vi "Calc Profile Data Size.vi"(4 "Profile Info":T1) -> (1 "Profile Data Size in U32":u32)   [LabVIEW 2014]
uses:
  Public/Clusters/Profile Info.ctl
  Keyence LJ-V7000.lvlib
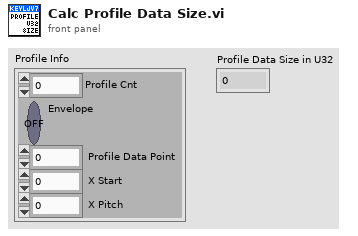
[diagram p1: front panel]
types:
  T1 = typedef "Keyence LJ-V7000.lvlib/Profile Info.ctl" = cluster{"Profile Cnt":u8, "Envelope":bool, " Profile Data Point":u16, " X Start":i32, " X Pitch":i32}
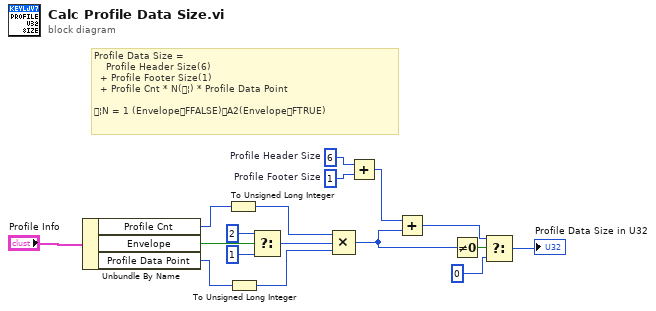
[diagram p0: block diagram]
diagram:
  w2 = u32 1  # Profile Footer Size
  w3 = u32 6  # Profile Header Size
  # "Profile Data Size =\n    Profile Header Size(6)\n  + Profile Footer Size(1)\n  + Profile Cnt * N(¦) * Profile Data Point\n\n¦N = 1 (EnvelopeFFALSE)A2(EnvelopeFTRUE)"
  n1 = Unbundle By Name("Profile Info") -> ("Profile Cnt"=w6:u8, "Envelope"=w5:bool, "Profile Data Point"=w4:u16)
  n2 = To Unsigned Long Integer(number=w6) -> (unsigned 32bit integer=w14:u32)
  n3 = To Unsigned Long Integer(number=w4) -> (unsigned 32bit integer=w12:u32)
  n4 = Select(t=u32 2, s=w5, f=u32 1) -> (s? t:f=w13:u32)
  n5 = Compound Arithmetic op=MULTIPLY(w14, w13, w12) -> (w9:u32)
  n6 = Add(x=w3, y=w2) -> (x+y=w11:u32)
  n7 = Add(x=w11, y=w9) -> (x+y=w8:u32)
  n8 = Not Equal To 0?(x=w9) -> (x != 0?=w10:bool)
  n9 = Select(t=w8, s=w10, f=u32 0) -> (s? t:f=→"Profile Data Size in U32":u32)
